vi "Test Arduino stepper API.vi"() -> ()   [LabVIEW 2020]
doc: "Arduino stepper API Tester."
uses:
  Support/COM params--typedef.ctl
  Support/Motor parameters.ctl
  <vilib>/Utility/error.llb/DialogType.ctl
  Arduino stepper.lvlib
panel:
  out "Connected?":bool
  in  "Read all info":bool
  out "End-stops":cluster{"ES1":bool, "ES2":bool}
  in  "Read end-stops":bool
  in  "Stop motor":bool
  out "End position?":bool
  out "String":string
  in  "Stop continuous reading":bool
  in  "Timeout":i32=100 format="%.0f ms"
  in  "Wake HL":bool
  out "Position":i32
  in  "Get position":bool
  in  "Move motor":bool
  in  "Motor params":T1={"Motor type"=enum."Unipolar", "Direction"=enum."CW", "Steps"=2048, "Frequency (Hz)"=255, "Step type"=enum."Full"}
  in  "Disconnect":bool
  in  "VISA resource":refnum<visa-resource-name>
  in  "COM params":T2={"baud rate"=115200, "data bits"=8, "parity"=enum."None", "stop bits"=10, "flow control"=0} {"stop bits" items=["1.0"=10, "1.5"=15, "2.0"=20]; "flow control" items=["None", "XON/XOFF", "RTS/CTS", "XON/XOFF & RTS/CTS", "DTR/DSR", "XON/XOFF & DTR/DSR"]}
  in  "Connect":bool
  in  "Show Diagram on Init":bool
  in  "Run as Singleton?":bool
  in  "Show Block Diagram":bool
  in  "Refresh Modules":bool
  out "Active Modules":string[](array[string])
  in  "Stop Module":bool
  in  "Select Module":i32(ring)=-1 caption="Select Module\nTo send Request to" items=["All"=-1, "1"=1]
  in  "Run New Module":bool
  in  "Hide Module Panel":bool
  in  "Show Module Panel":bool
  out "Status":string
  # "This VI tests the API for the Module."
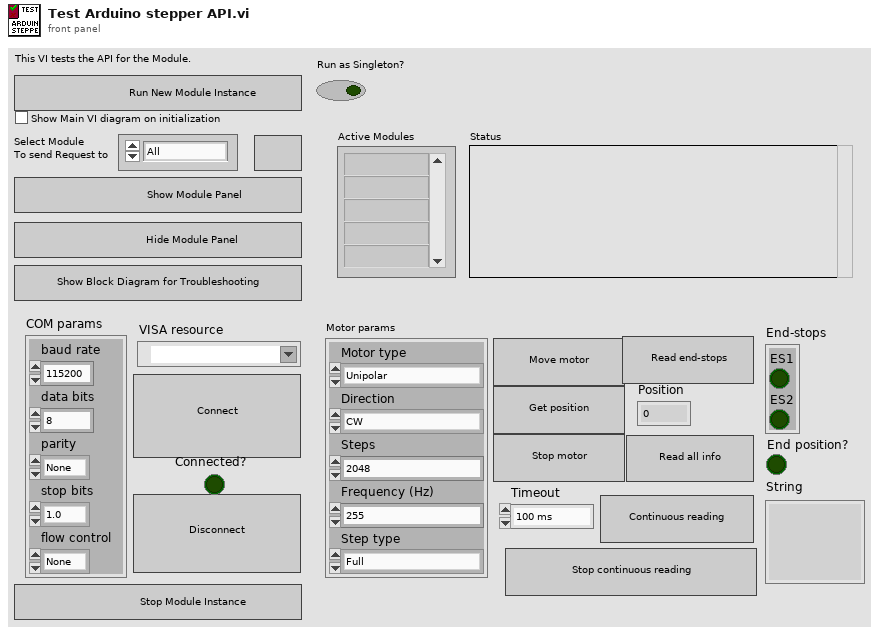
[diagram p1: front panel]
types:
  T1 = typedef "Arduino stepper.lvlib/Motor parameters.ctl" = cluster{"Motor type":enum8{"", "Unipolar", "Bipolar"}, "Direction":enum8{"", "CW", "CCW"}, "Steps":u16, "Frequency (Hz)":u8, "Step type":enum8{"", "Half", "Full"}}
  T2 = typedef "Arduino stepper.lvlib/COM params--typedef.ctl" = cluster{"baud rate":u32, "data bits":u16, "parity":enum16{"None", "Odd", "Even", "Mark", "Space"}, "stop bits":u16, "flow control":u16}
  T3 = typedef "Arduino stepper.lvlib/Broadcast Events--cluster.ctl" = cluster{"Module Did Init":refnum<user-event>, "Status Updated":refnum<user-event>, "Error Reported":refnum<user-event>, "Module Did Stop":refnum<user-event>, "Update Module Execution Status":refnum<user-event>, "Device connected":refnum<user-event>, "Data available":refnum<user-event>, "Info ready":refnum<user-event>, "Connection failed":refnum<user-event>, "Device disconected":refnum<user-event>}
  T4 = typedef "DialogType.ctl" = u16
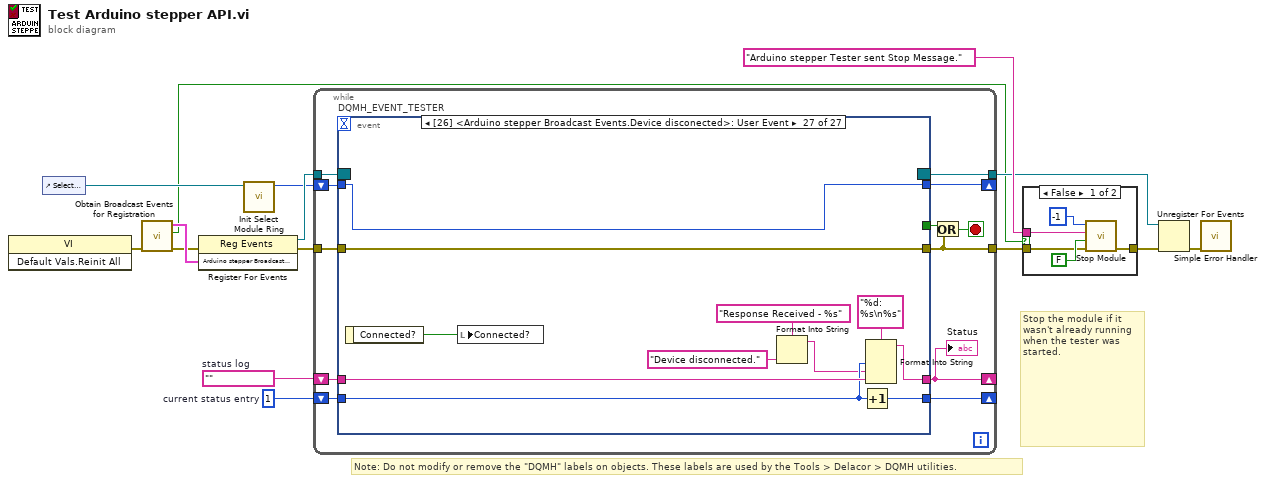
[diagram p0: block diagram]
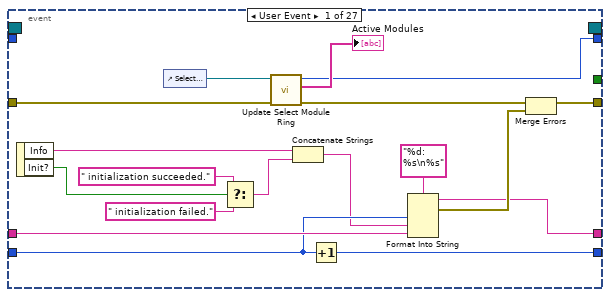
[diagram p3: hidden frame]
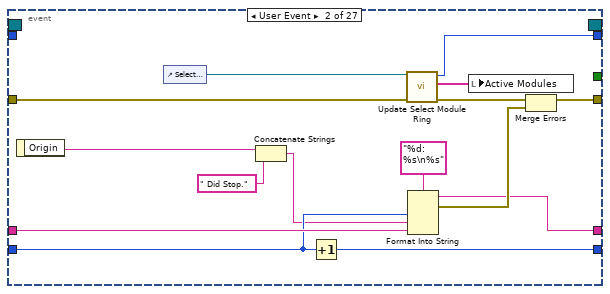
[diagram p4: hidden frame]
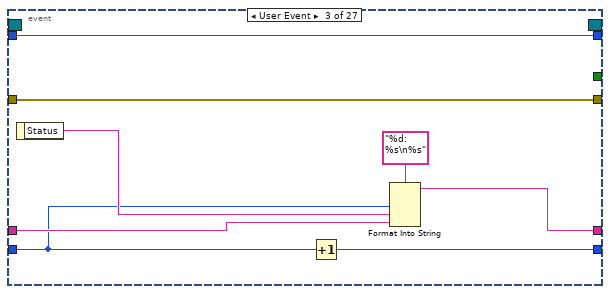
[diagram p5: hidden frame]
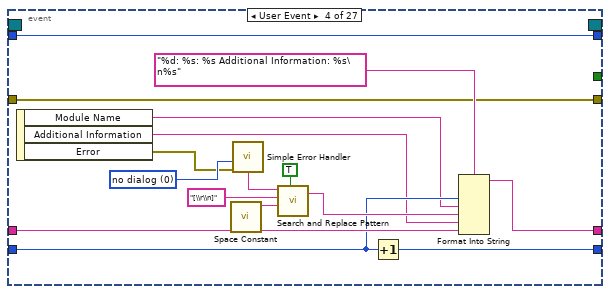
[diagram p6: hidden frame]
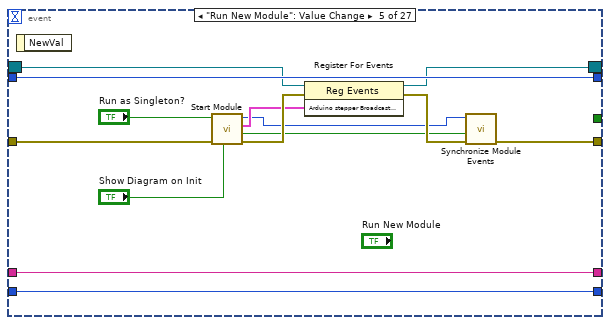
[diagram p7: hidden frame]
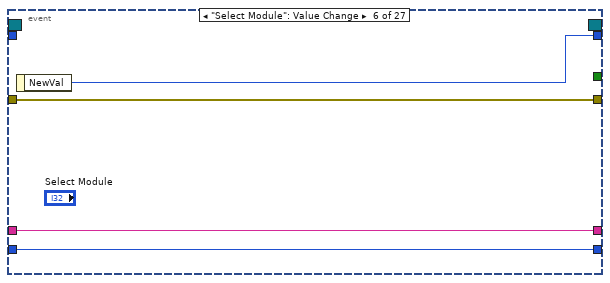
[diagram p8: hidden frame]
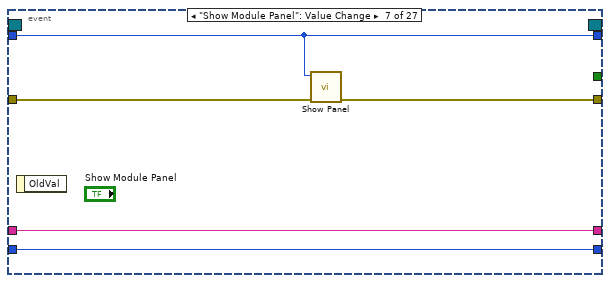
[diagram p9: hidden frame]
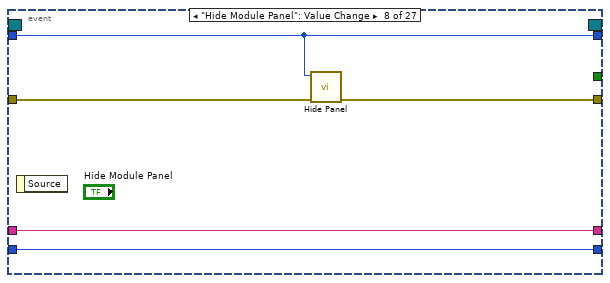
[diagram p10: hidden frame]
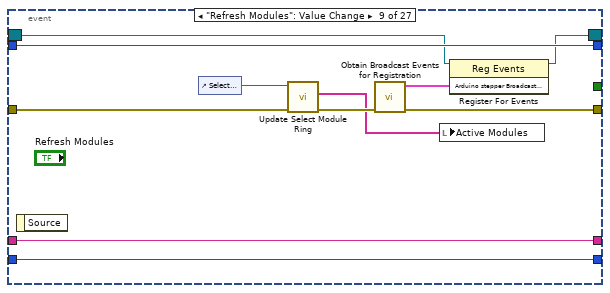
[diagram p11: hidden frame]
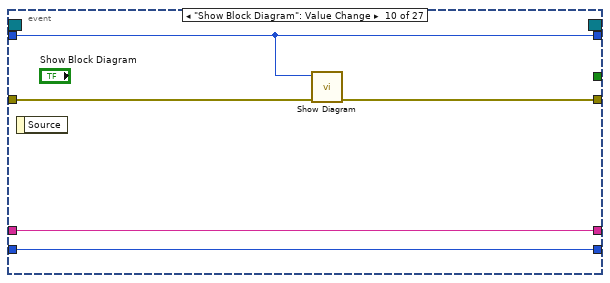
[diagram p12: hidden frame]
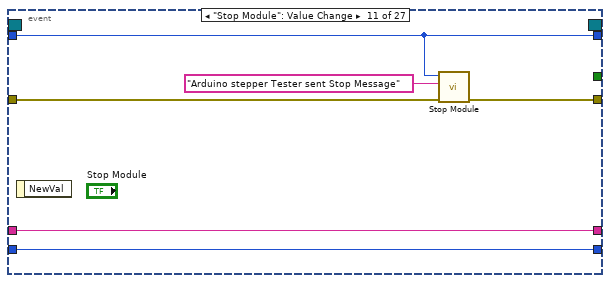
[diagram p13: hidden frame]
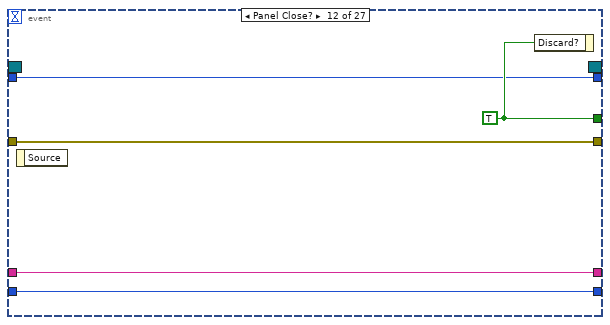
[diagram p14: hidden frame]
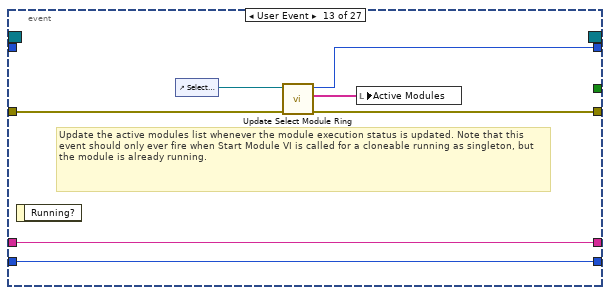
[diagram p15: hidden frame]
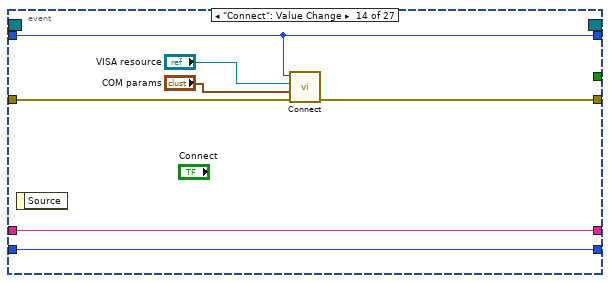
[diagram p16: hidden frame]
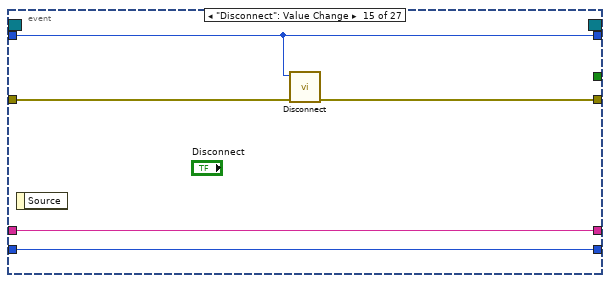
[diagram p17: hidden frame]
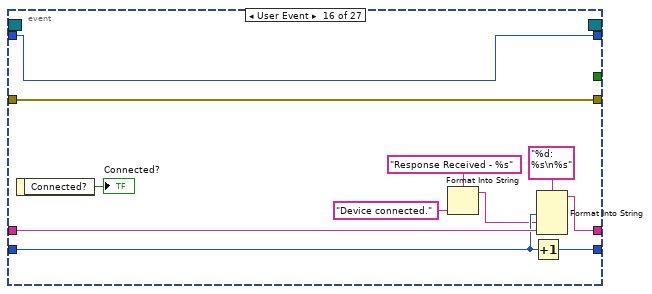
[diagram p18: hidden frame]
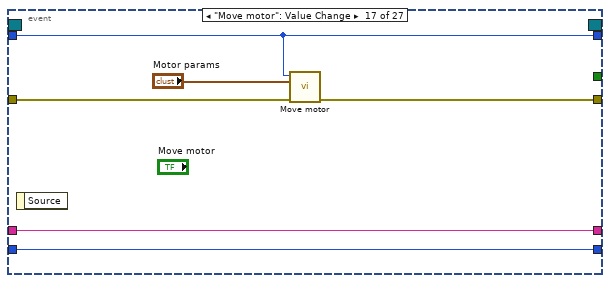
[diagram p19: hidden frame]
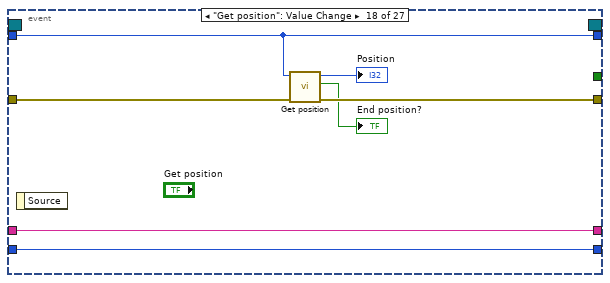
[diagram p20: hidden frame]
diagram:
  w12 = 1  # current status entry
  w13 = ""  # status log
  # "Stop the module if it wasn't already running when the tester was started."
  # "Note: Do not modify or remove the \"DQMH\" labels on objects. These labels are used by the Tools > Delacor > DQMH utilities."
  n1 = invoke class="VI" method="Default Vals.Reinit All"() -> (error out=w5:errorcluster)  [unwired: 3 in, 2 out]
  n2 = control-ref of="Select Module"() -> (w10:refnum<vi>)
  n3 = call "Obtain Broadcast Events for Registration.vi"("error in"=w5) -> ("error out"=w4:errorcluster, "Already running?"=w3:bool, "Arduino stepper Broadcast Events"=w9:T3)  [unwired: 8 in]
  n4 = register-events(error in=w4, w9) -> (reference out=w15:refnum<event-registration>, error out=w8:errorcluster)  [unwired: 1 in]
  n5 = call "Init Select Module Ring.vi"("Select Module Ring Ref"=w10) -> ("Value for All Modules"=w11:i32)  [unwired: 8 in, 2 out]
  n6 = while {
    tunnel: w15 -> [w27]
    tunnel: [w16] -> w2
    tunnel: w8 -> [w25]
    shift-right: [w21] -> _
    shift-left: w13 -> [w23]
    shift-right: [w22] -> _
    shift-left: w12 -> [w24]
    shift-right: [w18] -> _
    shift-left: w11 -> [w19]
    tunnel: [w17] -> w6
    stop <- w20 stop-if-true
    n7 = event "DQMH_EVENT_TESTER" shown="[26] <Arduino stepper Broadcast Events.Device disconected>: User Event" {
      selector: w27 -> [_ _ _ _ w92 _ _ _ w118 _ _ _ _ _ _ _ _ _ _ _ _ _ _ _ _ _ _]
      dyn-events: [_ _ _ _ w91 _ _ _ w117 _ _ _ _ _ _ _ _ _ _ _ _ _ _ _ _ _ _] -> w17
      timeout: _ -> [_ _ _ _ _ _ _ _ _ _ _ _ _ _ _ _ _ _ _ _ _ _ _ _ _ _ _]
      tunnel: [_ _ _ _ _ _ _ _ _ _ _ w139 _ _ _ _ _ _ _ _ _ _ _ _ _ _ _] -> w26
      tunnel: [w35 w52 w68 w72 w90 w102 w106 w111 w114 w125 w130 w138 w142 w150 w155 w169 w172 w179 w185 w190 w203 w205 w211 w216 w231 w242 w253] -> w16
      tunnel: w25 -> [w37 w54 w68 w72 w93 w102 w107 w112 w119 w128 w131 w138 w143 w153 w158 w169 w175 w182 w188 w193 w203 w208 w214 w219 w231 w242 w253]
      tunnel: w24 -> [w42 w57 w61 w75 w95 w100 w104 w109 w122 w126 w133 w136 w145 w151 w156 w165 w173 w180 w186 w191 w199 w206 w212 w217 w227 w238 w249]
      tunnel: w23 -> [w43 w58 w64 w76 w96 w101 w105 w110 w123 w127 w134 w137 w146 w152 w157 w167 w174 w181 w187 w192 w201 w207 w213 w218 w229 w240 w251]
      tunnel: [w40 w55 w65 w74 w96 w101 w105 w110 w123 w127 w134 w137 w146 w152 w157 w166 w174 w181 w187 w192 w200 w207 w213 w218 w228 w239 w250] -> w21
      tunnel: [w41 w56 w67 w73 w95 w100 w104 w109 w122 w126 w133 w136 w145 w151 w156 w164 w173 w180 w186 w191 w198 w206 w212 w217 w226 w237 w248] -> w22
      tunnel: w19 -> [_ _ w62 w84 w94 _ w103 w108 w121 w124 w132 w135 _ w149 w154 w168 w171 w178 w184 w189 w202 w204 w210 w215 w230 w241 w252]
      tunnel: [w32 w49 w62 w84 w94 w99 w103 w108 w121 w124 w132 w135 w141 w149 w154 w168 w171 w178 w184 w189 w202 w204 w210 w215 w230 w241 w252] -> w18
      event User Event {
        n8 = event-data() -> ("Info"=w39:string, "Init?"=w29:bool)  [unwired: 1 in]
        n9 = control-ref of="Select Module"() -> (w34:refnum<vi>)
        n10 = Select(t=" initialization succeeded.", s=w29, f=" initialization failed.") -> (s? t:f=w28:string)
        n11 = call "Update Select Module Ring.vi"("error in (no error)"=w37, "Select Module Ring Ref"=w34) -> ("error out"=w36:errorcluster, "Active Modules (Array)"=→"Active Modules":string[], "New Module Ring Value"=w32:i32)  [unwired: 7 in]
        n12 = Concatenate Strings(w39, w28) -> (w38:string)
        n13 = Increment(x=w42) -> (x+1=w41:i32)
        n14 = Format Into String(format string="%d: %s\n%s", w42, w38, w43) -> (resulting string=w40:string, error out=w45:errorcluster)  [unwired: 2 in]
        n15 = Merge Errors(w36, w45) -> (w35:errorcluster)
      }
      event User Event {
        n16 = event-data() -> ("Origin"=w47:string)  [unwired: 1 in]
        n17 = control-ref of="Select Module"() -> (w51:refnum<vi>)
        n18 = Concatenate Strings(w47, " Did Stop.") -> (w46:string)
        n19 = Increment(x=w57) -> (x+1=w56:i32)
        n20 = call "Update Select Module Ring.vi"("error in (no error)"=w54, "Select Module Ring Ref"=w51) -> ("error out"=w53:errorcluster, "Active Modules (Array)"=w50:string[], "New Module Ring Value"=w49:i32)  [unwired: 7 in]
        n21 = Format Into String(format string="%d: %s\n%s", w57, w46, w58) -> (resulting string=w55:string, error out=w60:errorcluster)  [unwired: 2 in]
        n22 = local write "Active Modules"(w50) -> ()
        n23 = Merge Errors(w53, w60) -> (w52:errorcluster)
      }
      event User Event {
        n24 = event-data() -> ("Status"=w63:string)  [unwired: 1 in]
        n25 = Increment(x=w61) -> (x+1=w67:i32)
        n26 = Format Into String(format string="%d: %s\n%s", w61, w63, w64) -> (resulting string=w65:string)  [unwired: 2 in, 1 out]
      }
      event User Event {
        w77 = T4 0 items=["no dialog", "OK message", "continue or stop message", "OK message + warnings", "continue/stop + warnings"] ("type of dialog (OK msg:1)")
        n27 = event-data() -> ("Module Name"=w71:string, "Additional Information"=w70:string, "Error"=w69:errorcluster)  [unwired: 1 in]
        n28 = call <vilib>:"Space Constant.vi"() -> ("String"=w81:string)
        n29 = call <vilib>:"Simple Error Handler.vi"("type of dialog (OK msg:1)"=w77, "error in (no error)"=w69) -> ("message"=w78:string)  [unwired: 3 in, 4 out]
        n30 = call <vilib>:"Search and Replace Pattern.vi"("string"=w78, "regular expression (\"\")"="[\\r\\n]" ("regular expression (\"\")"), "replace string (\"\")"=w81, "replace all? (F)"=TRUE ("replace all CR/LF with spaces")) -> ("result string"=w79:string)  [unwired: 1 in, 1 out]
        n31 = Increment(x=w75) -> (x+1=w73:i32)
        n32 = Format Into String(format string="%d: %s: %s Additional Information: %s\n%s", w75, w71, w79, w70, w76) -> (resulting string=w74:string)  [unwired: 2 in, 1 out]
      }
      event "Run New Module": Value Change {
        n33 = event-data() -> ()  [unwired: 1 in, 1 out]
        n34 = call "Start Module.vi"("Show Main VI Diagram on Init (F)"="Show Diagram on Init", "error in"=w93, "Run as Singleton? (F)"="Run as Singleton?") -> ("error out"=w97:errorcluster, "Wait for Event Sync?"=w89:bool, "Arduino stepper Broadcast Events"=w88:T3, "Module ID"=w85:i32)  [unwired: 5 in]
        n35 = register-events(reference=w92, error in=w97, w88) -> (reference out=w91:refnum<event-registration>, error out=w98:errorcluster)
        n36 = call "Synchronize Module Events.vi"("error in"=w98, "Wait for Event Sync?"=w89, "Module ID in"=w85) -> ("error out"=w90:errorcluster)  [unwired: 7 in, 1 out]
      }
      event "Select Module": Value Change {
        n37 = event-data() -> ("NewVal"=w99:i32)  [unwired: 1 in]
      }
      event "Show Module Panel": Value Change {
        n38 = event-data() -> ()  [unwired: 1 in, 1 out]
        n39 = call "Show Panel.vi"("error in (no error)"=w107, "Module ID"=w103) -> ("error out"=w106:errorcluster)  [unwired: 9 in]
      }
      event "Hide Module Panel": Value Change {
        n40 = event-data() -> ()  [unwired: 1 in, 1 out]
        n41 = call "Hide Panel.vi"("error in (no error)"=w112, "Module ID"=w108) -> ("error out"=w111:errorcluster)  [unwired: 9 in]
      }
      event "Refresh Modules": Value Change {
        n42 = event-data() -> ()  [unwired: 1 in, 1 out]
        n43 = control-ref of="Select Module"() -> (w120:refnum<vi>)
        n44 = call "Update Select Module Ring.vi"("error in (no error)"=w119, "Select Module Ring Ref"=w120) -> ("error out"=w115:errorcluster, "Active Modules (Array)"=w113:string[])  [unwired: 7 in, 1 out]
        n45 = call "Obtain Broadcast Events for Registration.vi"("error in"=w115) -> ("error out"=w114:errorcluster, "Arduino stepper Broadcast Events"=w116:T3)  [unwired: 8 in, 1 out]
        n46 = local write "Active Modules"(w113) -> ()
        n47 = register-events(reference=w118, w116) -> (reference out=w117:refnum<event-registration>)  [unwired: 1 in, 1 out]
      }
      event "Show Block Diagram": Value Change {
        n48 = event-data() -> ()  [unwired: 1 in, 1 out]
        n49 = call "Show Diagram.vi"("error in (no error)"=w128, "Module ID"=w124) -> ("error out"=w125:errorcluster)  [unwired: 9 in]
      }
      event "Stop Module": Value Change {
        n50 = event-data() -> ()  [unwired: 1 in, 1 out]
        n51 = call "Stop Module.vi"("error in"=w131, "Origin"="Arduino stepper Tester sent Stop Message", "Module ID"=w132) -> ("error out"=w130:errorcluster)  [unwired: 8 in]
      }
      event Panel Close? {
        w139 = TRUE ("Discard?")
        n52 = event-data() -> ()  [unwired: 1 in, 1 out]
        n53 = event-data("Discard?"=w139) -> ()  [unwired: 1 in, 1 out]
      }
      event User Event {
        # "Update the active modules list whenever the module execution status is updated. Note that this event should only ever fire when Start Module VI is called for a cloneable running as singleton, but the module is already running."
        n54 = event-data() -> ()  [unwired: 1 in, 1 out]
        n55 = control-ref of="Select Module"() -> (w144:refnum<vi>)
        n56 = call "Update Select Module Ring.vi"("error in (no error)"=w143, "Select Module Ring Ref"=w144) -> ("error out"=w142:errorcluster, "Active Modules (Array)"=w140:string[], "New Module Ring Value"=w141:i32)  [unwired: 7 in]
        n57 = local write "Active Modules"(w140) -> ()
      }
      event "Connect": Value Change {
        n58 = event-data() -> ()  [unwired: 1 in, 1 out]
        n59 = call "Connect.vi"("error in"=w153, "COM params"="COM params", "VISA resource"="VISA resource", "Module ID"=w149) -> ("error out"=w150:errorcluster)  [unwired: 7 in]
      }
      event "Disconnect": Value Change {
        n60 = event-data() -> ()  [unwired: 1 in, 1 out]
        n61 = call "Disconnect.vi"("error in"=w158, "Module ID"=w154) -> ("error out"=w155:errorcluster)  [unwired: 9 in]
      }
      event User Event {
        n62 = event-data() -> ("Connected?"=→"Connected?":bool)  [unwired: 1 in]
        n63 = Format Into String(format string="Response Received - %s", "Device connected." ("input 1")) -> (resulting string=w161:string)  [unwired: 2 in, 1 out]
        n64 = Increment(x=w165) -> (x+1=w164:i32)
        n65 = Format Into String(format string="%d: %s\n%s", w165, w161, w167) -> (resulting string=w166:string)  [unwired: 2 in, 1 out]
      }
      event "Move motor": Value Change {
        n66 = event-data() -> ()  [unwired: 1 in, 1 out]
        n67 = call "Move motor.vi"("error in"=w175, "Motor params"="Motor params", "Module ID"=w171) -> ("error out"=w172:errorcluster)  [unwired: 8 in]
      }
      event "Get position": Value Change {
        n68 = event-data() -> ()  [unwired: 1 in, 1 out]
        n69 = call "Get position.vi"("error in"=w182, "Module ID"=w178) -> ("error out"=w179:errorcluster, "End position?"=→"End position?":bool, "Position"=→"Position":i32)  [unwired: 6 in, 1 out]
      }
      event "Wake HL": Value Change {
        n70 = event-data() -> ()  [unwired: 1 in, 1 out]
        n71 = call "Read port continuously.vi"("error in"=w188, "Timeout"="Timeout", "Module ID"=w184) -> ("error out"=w185:errorcluster)  [unwired: 8 in]
      }
      event "Stop continuous reading": Value Change {
        n72 = event-data() -> ()  [unwired: 1 in, 1 out]
        n73 = call "Stop continuous reading.vi"("error in"=w193, "Module ID"=w189) -> ("error out"=w190:errorcluster)  [unwired: 9 in]
      }
      event User Event {
        n74 = event-data() -> ("Data"=w194:string)  [unwired: 1 in]
        "String" <- w194
        n75 = Format Into String(format string="Response Received - %s", w194) -> (resulting string=w195:string)  [unwired: 2 in, 1 out]
        n76 = Increment(x=w199) -> (x+1=w198:i32)
        n77 = Format Into String(format string="%d: %s\n%s", w199, w195, w201) -> (resulting string=w200:string)  [unwired: 2 in, 1 out]
      }
      event "Stop motor": Value Change {
        n78 = event-data() -> ()  [unwired: 1 in, 1 out]
        n79 = call "Stop motor.vi"("error in"=w208, "Module ID"=w204) -> ("error out"=w205:errorcluster)  [unwired: 9 in]
      }
      event "Read end-stops": Value Change {
        n80 = event-data() -> ()  [unwired: 1 in, 1 out]
        n81 = call "Read end-stops.vi"("error in"=w214, "Module ID"=w210) -> ("error out"=w211:errorcluster, "End-stops"=→"End-stops":cluster{"ES1":bool, "ES2":bool})  [unwired: 7 in, 1 out]
      }
      event "Read all info": Value Change {
        n82 = event-data() -> ()  [unwired: 1 in, 1 out]
        n83 = call "Read all info.vi"("error in"=w219, "Module ID"=w215) -> ("error out"=w216:errorcluster)  [unwired: 9 in]
      }
      event User Event {
        n84 = event-data() -> ("Position"=w220:i32, "End-stops"=w221:cluster{"ES1":bool, "ES2":bool})  [unwired: 1 in]
        n85 = local write "End-stops"(w221) -> ()
        n86 = local write "Position"(w220) -> ()
        n87 = Format Into String(format string="Response Received - %s", "Info ready.." ("input 1")) -> (resulting string=w223:string)  [unwired: 2 in, 1 out]
        n88 = Increment(x=w227) -> (x+1=w226:i32)
        n89 = Format Into String(format string="%d: %s\n%s", w227, w223, w229) -> (resulting string=w228:string)  [unwired: 2 in, 1 out]
      }
      event User Event {
        n90 = event-data() -> ("Connected?"=w232:bool)  [unwired: 1 in]
        n91 = local write "Connected?"(w232) -> ()
        n92 = Format Into String(format string="Response Received - %s", "Connection failed." ("input 1")) -> (resulting string=w234:string)  [unwired: 2 in, 1 out]
        n93 = Increment(x=w238) -> (x+1=w237:i32)
        n94 = Format Into String(format string="%d: %s\n%s", w238, w234, w240) -> (resulting string=w239:string)  [unwired: 2 in, 1 out]
      }
      event User Event {
        n95 = event-data() -> ("Connected?"=w243:bool)  [unwired: 1 in]
        n96 = local write "Connected?"(w243) -> ()
        n97 = Format Into String(format string="Response Received - %s", "Device disconnected." ("input 1")) -> (resulting string=w245:string)  [unwired: 2 in, 1 out]
        n98 = Increment(x=w249) -> (x+1=w248:i32)
        n99 = Format Into String(format string="%d: %s\n%s", w249, w245, w251) -> (resulting string=w250:string)  [unwired: 2 in, 1 out]
      }
    }
    "Status" <- w21
    n100 = Or(x=w26, y=w16) -> (x .or. y?=w20:bool)
  }
  n101 = case shown="False" w3 {
    tunnel: [w258 w259] -> w14
    tunnel: "Arduino stepper Tester sent Stop Message." ("Origin") -> [w257 _]
    tunnel: w2 -> [w254 w259]
    frame False {
      n102 = call "Stop Module.vi"("error in"=w254, "Wait for Module to stop? (F)"=FALSE ("Wait for Module to stop?"), "Origin"=w257, "Module ID"=-1 ("Stop all")) -> ("error out"=w258:errorcluster)  [unwired: 7 in]
    }
    frame True {
    }
  }
  n103 = Unregister For Events(event registration refnum=w6, error in=w14) -> (error out=w1:errorcluster)
  n104 = call <vilib>:"Simple Error Handler.vi"("error in (no error)"=w1) -> ()  [unwired: 4 in, 5 out]
